vi "Equip-Set Slot Controls.vi"(0 "connector types":T1[](array[typedef]), 7 "Slot Num":u32[](array[numeric]), 9 "slot ctl refs":refnum<vi>[](array[refnum]), 11 "error in (no error)":errorcluster, 12 "Trigger Slot":i32) -> (10 "slot ctl refs out":refnum<vi>[](array[refnum]), 15 "error out":errorcluster)   [LabVIEW 2020]
uses:
  Type Defs/PXISlot XControl/Connector Type.ctl
  Type Defs/PXISlot XControl/PXISlot.xctl
  Type Defs/Output sources.ctl
  Type Defs/Input sources.ctl
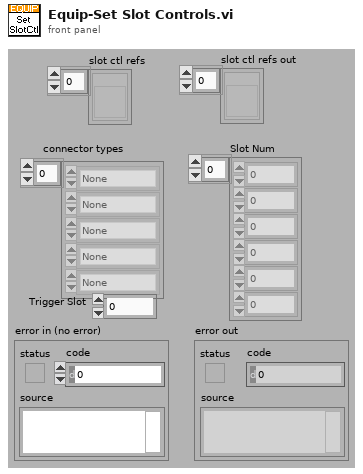
[diagram p1: front panel]
types:
  T1 = typedef "Connector Type.ctl" = enum16{"None", "PXI-4461", "BNC-2110", "BNC-2090", "PXIe-4463", "PXIe-4464"}
  T2 = typedef "Output sources.ctl" = u16
  T3 = typedef "Input sources.ctl" = u16
  T4 = cluster{"Output sources":T2[], "Input sources":T3[]}
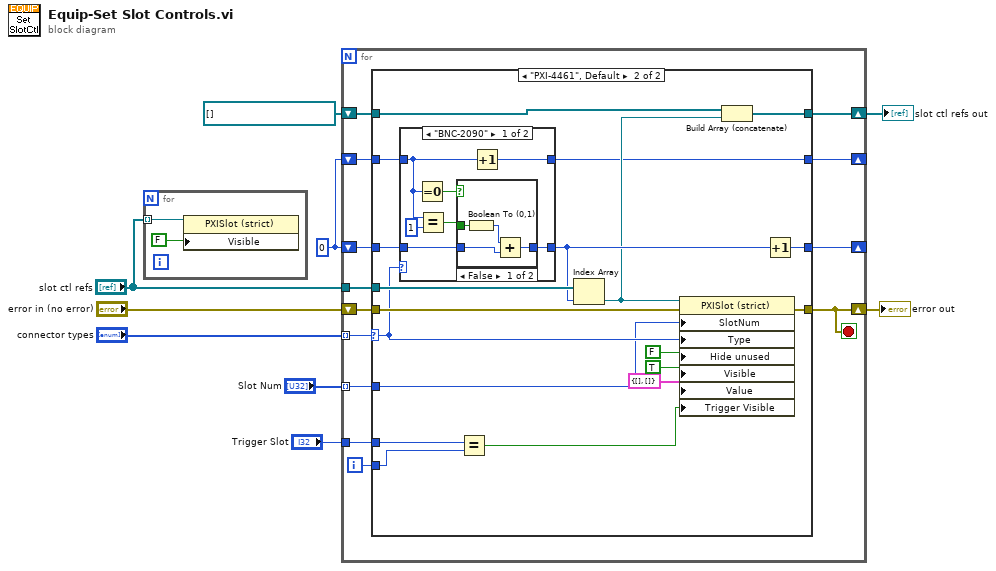
[diagram p0: block diagram]
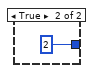
[diagram p3: hidden frame]
diagram:
  w3 = 0
  n1 = for {
    tunnel: "slot ctl refs" -> [w11] mode=indexing
    n2 = property class="PXISlot (strict)"(reference=w11, "Visible"=FALSE) -> ()  [unwired: 1 in, 2 out]
  }
  n3 = for {
    tunnel: "slot ctl refs" -> [w23]
    shift-right: [w12] -> w7
    shift-left: "error in (no error)" -> [w24]
    tunnel: "connector types" -> [w20] mode=indexing
    shift-right: [w21] -> _
    shift-left: w3 -> [w22]
    shift-right: [w19] -> w5
    shift-left: refnum<vi>[] [] -> [w18]
    shift-right: [w15] -> _
    shift-left: w3 -> [w16]
    tunnel: "Trigger Slot" -> [w14]
    tunnel: "Slot Num" -> [w13] mode=indexing
    i -> [w17]
    stop <- w12 stop-if-true
    n4 = case shown="\"PXI-4461\", Default" w20 {
      selector: w20 -> [_ w32]
      tunnel: w24 -> [w27 w47]
      tunnel: [w27 w46] -> w12
      tunnel: w23 -> [_ w42]
      tunnel: w22 -> [w28 w41]
      tunnel: [w28 w40] -> w21
      tunnel: [w26 w37] -> w19
      tunnel: w18 -> [w26 w36]
      tunnel: w17 -> [_ w29]
      tunnel: w16 -> [w25 w35]
      tunnel: [w25 w34] -> w15
      tunnel: w14 -> [_ w30]
      tunnel: w13 -> [_ w31]
      frame "None" {
      }
      frame "PXI-4461", Default {
        n5 = case shown="\"BNC-2090\"" w32 {
          tunnel: w41 -> [w54 w61]
          tunnel: [w53 w61] -> w39
          tunnel: w35 -> [w49 w60]
          tunnel: [w51 w60] -> w34
          frame "BNC-2090" {
            n6 = Equal To 0?(x=w49) -> (x = 0?=w52:bool)
            n7 = Equal?(x=w49, y=1) -> (x = y?=w50:bool)
            n8 = case shown="False" w52 {
              tunnel: w54 -> [w57 _]
              tunnel: [w58 2] -> w53
              tunnel: w50 -> [w55 _]
              frame False {
                n9 = Boolean To (0,1)(Boolean=w55) -> (0, 1=w56:i16)
                n10 = Add(x=w56, y=w57) -> (x+y=w58:i32)
              }
              frame True {
              }
            }
            n11 = Increment(x=w49) -> (x+1=w51:i32)
          }
          frame "PXI-4461", Default {
          }
        }
        n12 = Equal?(x=w30, y=w29) -> (x = y?=w33:bool)
        n13 = Index Array(array=w42, index=w39) -> (element=w38:refnum<vi>)
        n14 = property class="PXISlot (strict)"(reference=w38, error in=w47, "SlotNum"=w31, "Type"=w32, "Hide unused"=FALSE, "Visible"=TRUE, "Value"=T4 {"Output sources"=[], "Input sources"=[]}, "Trigger Visible"=w33) -> (error out=w46:errorcluster)  [unwired: 1 out]
        n15 = Build Array (concatenate)(w36, w38) -> (w37:refnum<vi>[])
        n16 = Increment(x=w39) -> (x+1=w40:i32)
      }
    }
  }
  "error out" <- w7
  "slot ctl refs out" <- w5
